vi "CMN_PassMsgToRunProc.vi"(7 "VItoRun":path, 11 "error in (no error)":errorcluster, 12 "Wait Until Done":bool) -> (6 "Result":string, 15 "error out":errorcluster)   [LabVIEW 2016]
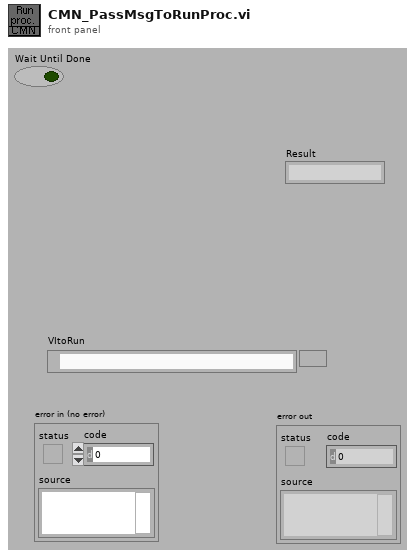
[diagram p1: front panel]
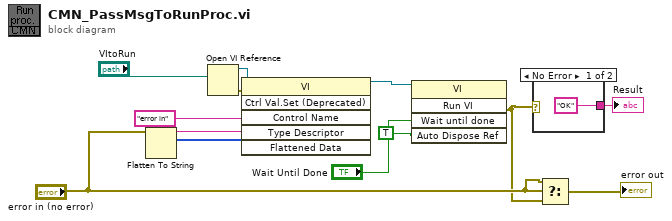
[diagram p0: block diagram]
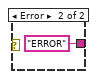
[diagram p2: hidden frame]
diagram:
  n1 = Flatten To String(anything="error in (no error)") -> (data string=w8:string, type string=w9:i16[])  [unwired: 1 in, 3 out]
  n2 = Open VI Reference(vi path="VItoRun") -> (vi reference=w12:refnum<vi>, error out=w11:errorcluster)  [unwired: 2 in, 3 out]
  n3 = invoke class="VI" method="Ctrl Val.Set (Deprecated)"(reference=w12, error in=w11, "Control Name"="error in" ("control\nname"), "Type Descriptor"=w9, "Flattened Data"=w8) -> (reference out=w7:refnum<vi>)  [unwired: 1 in, 5 out]
  n4 = invoke class="VI" method="Run VI"(reference=w7, "Wait until done"="Wait Until Done", "Auto Dispose Ref"=TRUE ("Auto Dispose Reference")) -> (error out=w2:errorcluster)  [unwired: 2 in, 4 out]
  n5 = case shown="No Error" w2 {
    tunnel: ["OK" ("queue element") "ERROR" ("queue element")] -> w13
    frame No Error {
    }
    frame Error {
    }
  }
  "Result" <- w13
  n6 = Select(t="error in (no error)", s="error in (no error)", f=w2) -> (s? t:f=→"error out":errorcluster)
